vi "userinterface page 1.vi"() -> ()   [LabVIEW 2023]
panel:
  out "Boolean":bool
  out "String 3":string
  out "String 2":string
  out "String":string
  out "Kickdown":string
  out "Engine Hour":string
  out "Fuel Level":string
  in  "Blank Button 15":bool
  in  "Blank Button 14":bool
  in  "Blank Button 13":bool
  in  "Blank Button 12":bool
  in  "Blank Button 11":bool
  in  "Blank Button 10":bool
  in  "Blank Button 9":bool
  in  "Blank Button 8":bool
  in  "Blank Button 7":bool
  in  "Blank Button 6":bool
  in  "Blank Button 5":bool
  in  "Blank Button 4":bool
  out "Blank Button 3":bool
  out "led 1":bool
  out "Tcs Voltage":dbl(knob) scale=0.0..40.0
  in  "Coolant Temperature":dbl(knob) scale=0.0..120.0 scale format="%#.7g"
  in  "Oil Pressure":dbl(knob) scale=1.0..5.0 scale format="%#.6g"
  # "Bar"
  # "Deg C"
  # "Volt"
  # "Start Lock"
  # "Batt Not Charge"
  # "Oil Pressure"
  # "Fording"
  # "Coolant Temp"
  # "Kick Down"
  # "Coolant Level 1"
  # "Litres"
  # "Air Filter"
  # "Coolant Level 2"
  # "Air Filter A"
  # "Coolant Circuit Control"
  # "Air Filter B"
  # "Dust Blower A"
  # "Emergency Shut Down"
  # "Dust Blower B"
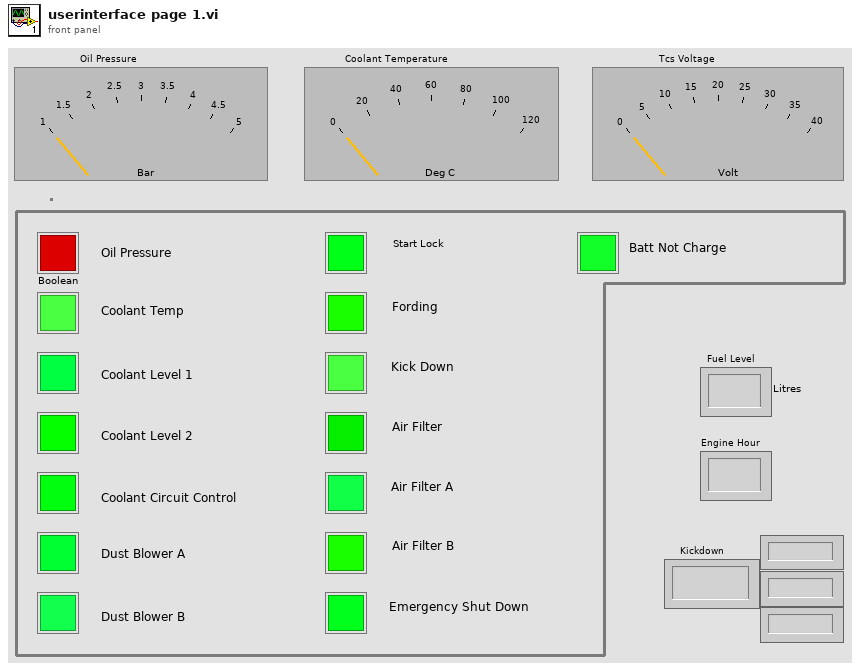
[diagram p1: front panel]
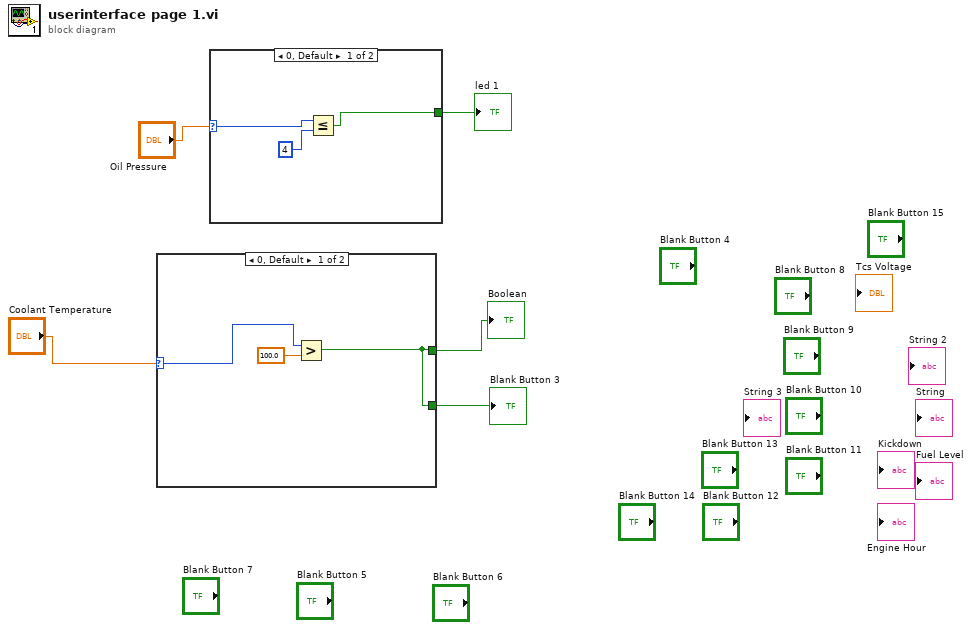
[diagram p0: block diagram]
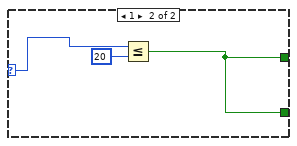
[diagram p2: hidden frame]
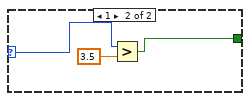
[diagram p3: hidden frame]
diagram:
  n1 = case shown="0, Default" "Coolant Temperature" {
    selector: "Coolant Temperature" -> [w7 w11]
    tunnel: [w6 w9] -> w2
    tunnel: [w6 w9] -> w1
    frame 0, Default {
      n2 = Greater?(x=w7, y=100.0) -> (0:w6:bool)
    }
    frame 1 {
      n3 = Less Or Equal?(x=w11, y=20) -> (x <= y?=w9:bool)
    }
  }
  "Blank Button 3" <- w1
  "Boolean" <- w2
  n4 = case shown="0, Default" "Oil Pressure" {
    selector: "Oil Pressure" -> [w14 w15]
    tunnel: [w12 w16] -> w5
    frame 0, Default {
      n5 = Less Or Equal?(x=w14, y=4) -> (x <= y?=w12:bool)
    }
    frame 1 {
      n6 = Greater?(x=w15, y=3.5) -> (0:w16:bool)
    }
  }
  "led 1" <- w5
